vi "saveSettings.vi"(8 "error in (no error)":errorcluster, 11 "Settings in":refnum<class "Settings.lvclass">) -> (0 "error out":errorcluster, 3 "Settings out":refnum<class "Settings.lvclass">)   [LabVIEW 2016, in "Settings.lvclass"]
uses:
  Settings.lvclass
  Settings.lvclass/Settings.ctl
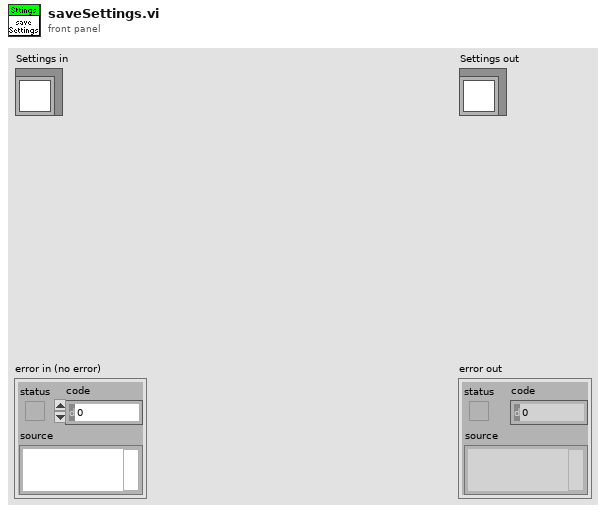
[diagram p1: front panel]
types:
  T1 = enum16{"open", "replace", "create", "open or create", "replace or create", "replace or create with confirmation"}
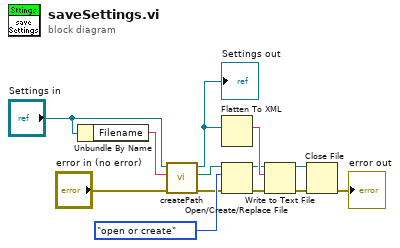
[diagram p0: block diagram]
diagram:
  n1 = Unbundle By Name("Settings in") -> ("Filename"=w13:string)
  n2 = call "createPath.vi"("error in (no error)"="error in (no error)", "filename"=w13, "Settings in"="Settings in") -> ("error out"=w9:errorcluster, "Path"=w8:path, "Settings out"=w7:refnum<class "Settings.lvclass">)  [unwired: 6 in]
  "Settings out" <- w7
  n3 = Flatten To XML(anything=w7) -> (xml string=w5:string)
  n4 = Open/Create/Replace File(file path (use dialog)=w8, error in=w9, operation (0:open)=T1."open or create") -> (refnum out=w4:refnum<file>, error out=w3:errorcluster)  [unwired: 3 in, 1 out]
  n5 = Write to Text File(file (use dialog)=w4, text=w5, error in=w3) -> (refnum out=w1:refnum<file>, error out=w2:errorcluster)  [unwired: 1 in, 1 out]
  n6 = Close File(refnum=w1, error in=w2) -> (error out=→"error out":errorcluster)  [unwired: 1 out]
